vi "4461 - Create IO Channels Parallel.vi"(6 "error in":errorcluster, 7 "AI Buffer Size (S)":i32=10, 8 "sampling info":cluster{"Fs":dbl, "#s":dbl}, 9 "AO":T1={"AO amp (V)"=[0.1, 0.09, 0.08, 0.07, 0.06, 0.05, 0.04, 0.03], "AO DC (V)"=[0.0, 0.0, 0.0, 0.0, 0.0, 0.0, 0.0, 0.0], "AO f (Hz)"=[13.0, 13.0, 13.0, 13.0, 13.0, 13.0, 13.0, 13.0], "AO phi (deg)"=[0.0, 0.0, 0.0, 0.0, 0.0, 0.0, 0.0, 0.0], "function"=[enum."Sine Wave", enum."Sine Wave", enum."Sine Wave", enum."Sine Wave", enum."Sine Wave", enum."Sine Wave", enum."Sine Wave", enum."Sine Wave"]} {"AO DC (V)" format="%#_6p"; "AO amp (V)" format="%#_6p"}, 10 "AO Configuration":T2(array[cluster])=[{"Output physical channels"="PXI1Slot2/ao0", "AO. Max"=0.1, "AO.Min"=-0.1}, {"Output physical channels"="", "AO. Max"=0.1, "AO.Min"=-0.1}], 11 "AI Configuration":T3(array[cluster])=[{"AI.Coupling"=10050, "AI.Max"=10.0, "AI.Min"=-10.0, "Input physical channels"="PXI1Slot2/ai0:1"}, {"AI.Coupling"=10050, "AI.Max"=10.0, "AI.Min"=-10.0, "Input physical channels"="PXI1Slot3/ai0:3"}, {"AI.Coupling"=10050, "AI.Max"=10.0, "AI.Min"=-10.0, "Input physical channels"=""}] {"AI.Coupling" items=["AC"=10045, "DC"=10050, "GND"=10066]}) -> (2 "AO Task":refnum<k21>[](array[refnum]), 3 "AI task":refnum<k21>[](array[refnum]), 4 "error out":errorcluster, 5 "phase log":dbl[](array[numeric])=[0.99999999999938, 0.99999999999938])   [LabVIEW 2013]
uses:
  <vilib>/DAQmx/write.llb/DAQmx Write (Analog 1D Wfm NChan NSamp).vi
  <vilib>/DAQmx/create/channels.llb/DAQmx Create Channel (AO-Voltage-Basic).vi
  <vilib>/DAQmx/configure/timing.llb/DAQmx Timing (Sample Clock).vi
  <vilib>/DAQmx/create/channels.llb/DAQmx Create Channel (AI-Voltage-Basic).vi
  <vilib>/DAQmx/configure/trigger.llb/DAQmx Start Trigger (Digital Edge).vi
  <vilib>/DAQmx/miscellaneous.llb/DAQmx Fill In Error Info.vi
  <resource>/objmgr/daqmx.rc
panel:
  out "AI.Gain":dbl
  in  "input terminal configuration":i32(ring)=-1 items=["default"=-1, "RSE"=10083, "NRSE"=10078, "Differential"=10106, "Pseudodifferential"=12529]
  in  "output terminal configuration":i32(ring)=-1 items=["Default"=-1, "RSE"=10083, "Differential"=10106, "Pseudodifferential"=12529]
  out "SampClk.Timebase.Rate":dbl
  out "SampQuant.SampPerChan":dbl
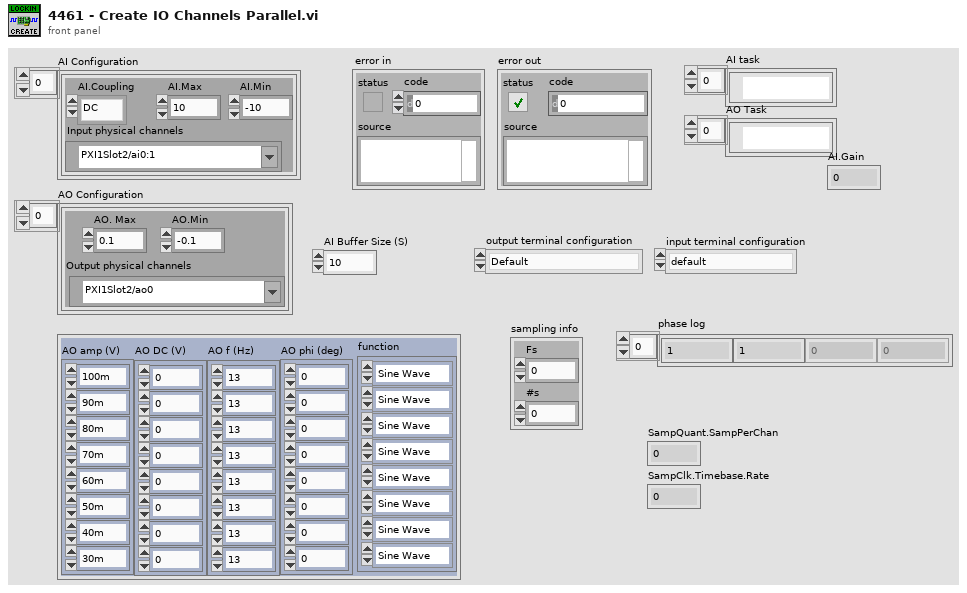
[diagram p1: front panel]
types:
  T1 = cluster{"AO amp (V)":dbl[], "AO DC (V)":dbl[], "AO f (Hz)":dbl[], "AO phi (deg)":dbl[], "function":enum16{"Sine Wave", "Triangle Wave", "Square Wave", "Sawtooth Wave"}[]}
  T2 = cluster{"Output physical channels":tag, "AO. Max":dbl, "AO.Min":dbl}[]
  T3 = cluster{"AI.Coupling":i32, "AI.Max":dbl, "AI.Min":dbl, "Input physical channels":tag}[]
  T4 = cluster{"AI.Coupling":i32, "AI.Max":dbl, "AI.Min":dbl, "Input physical channels":tag}
  T5 = cluster{"Output physical channels":tag, "AO. Max":dbl, "AO.Min":dbl}
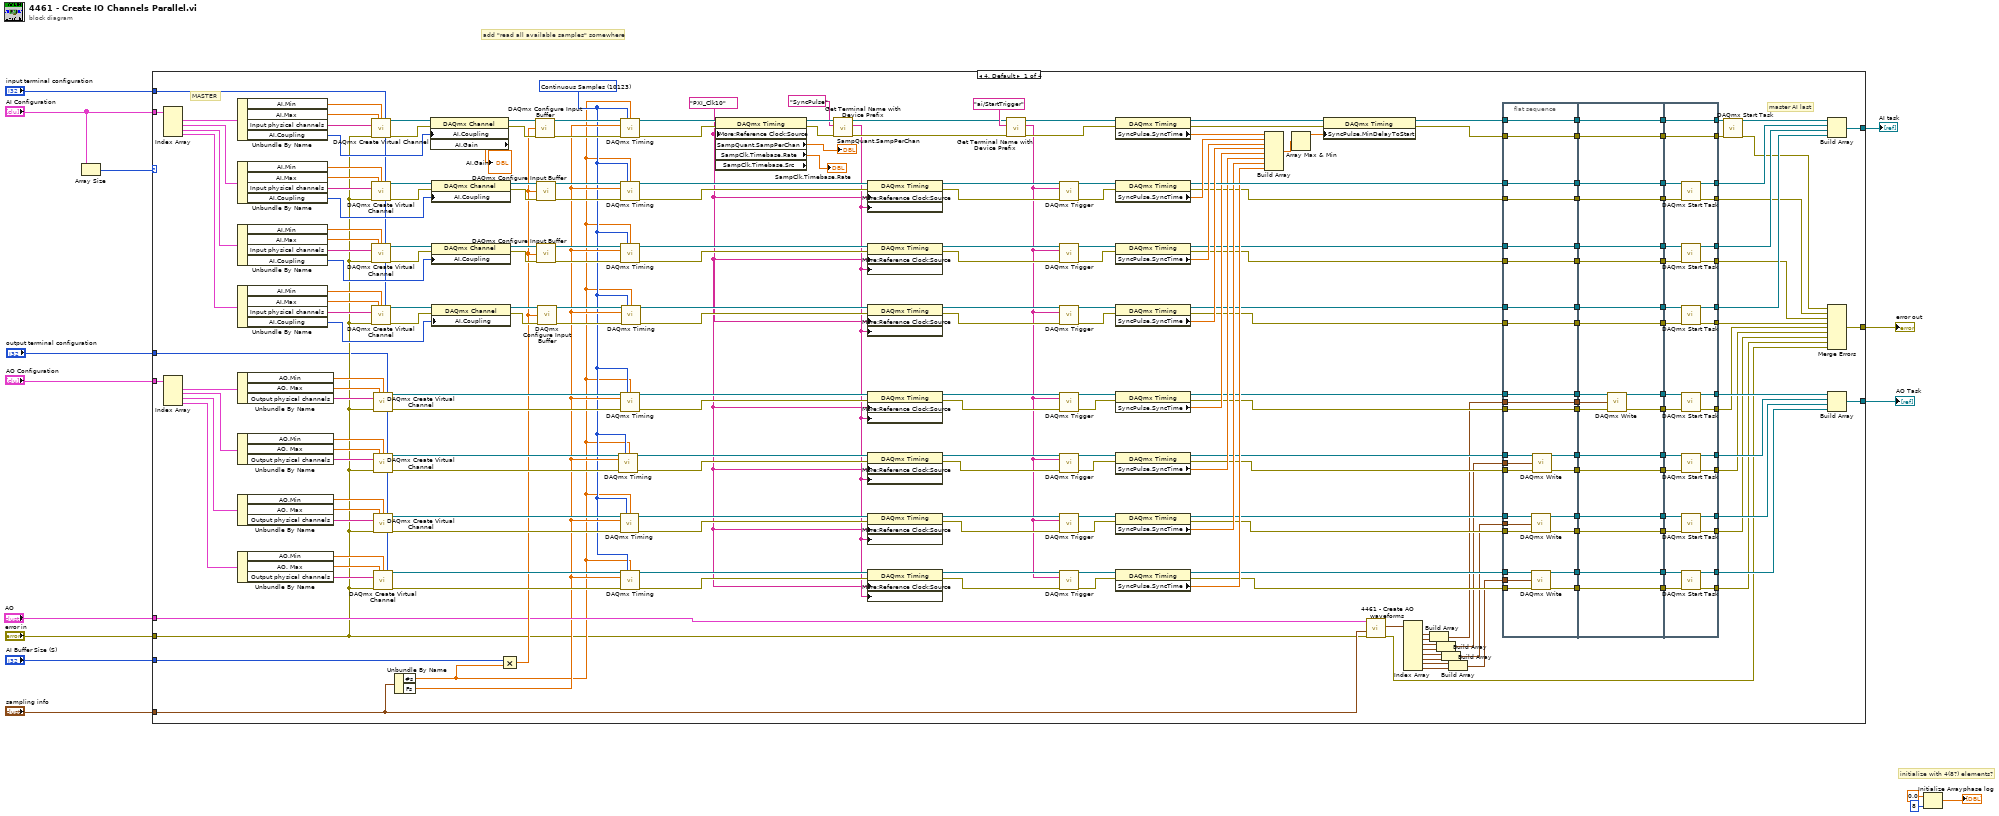
[diagram p0: block diagram]
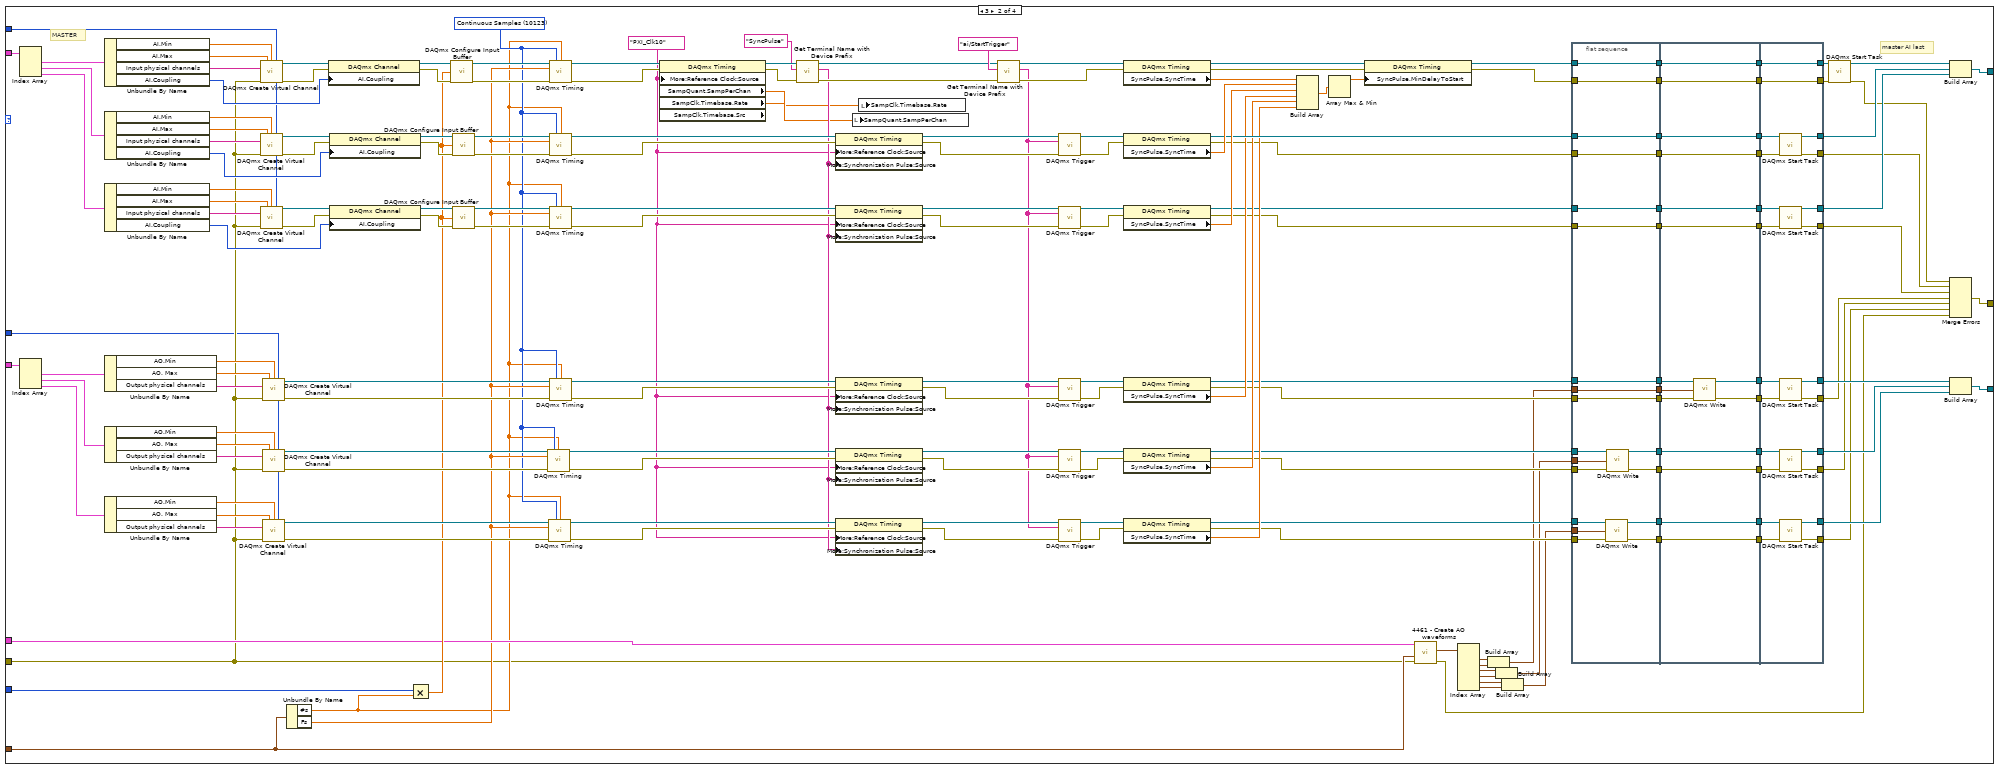
[diagram p2: hidden frame]
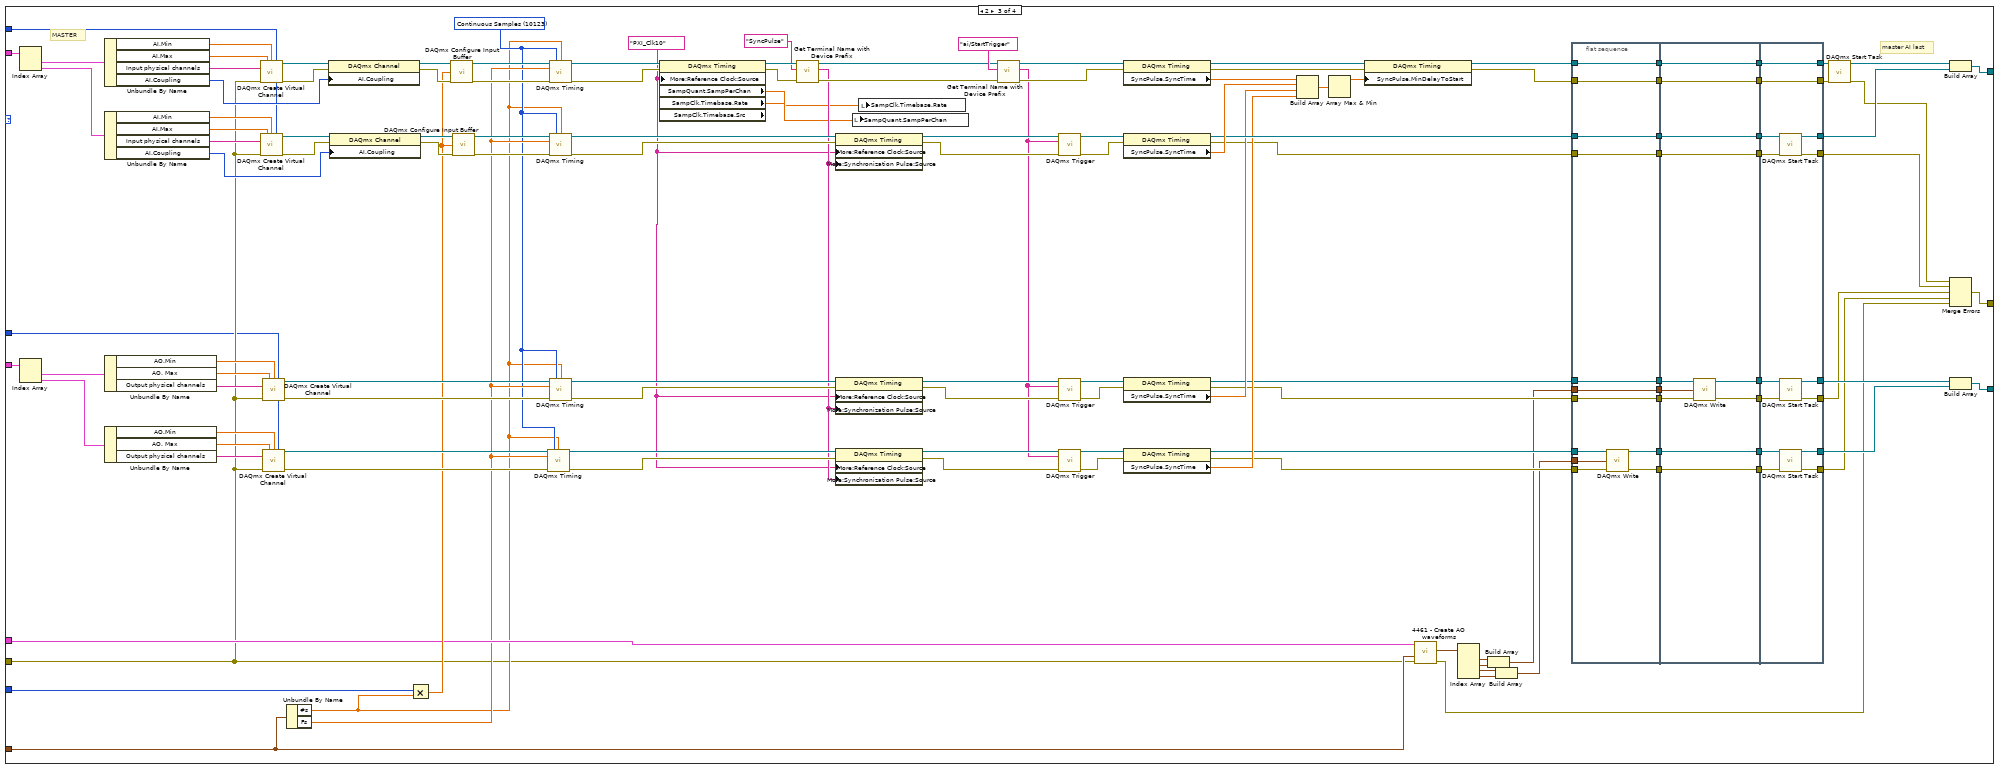
[diagram p3: hidden frame]
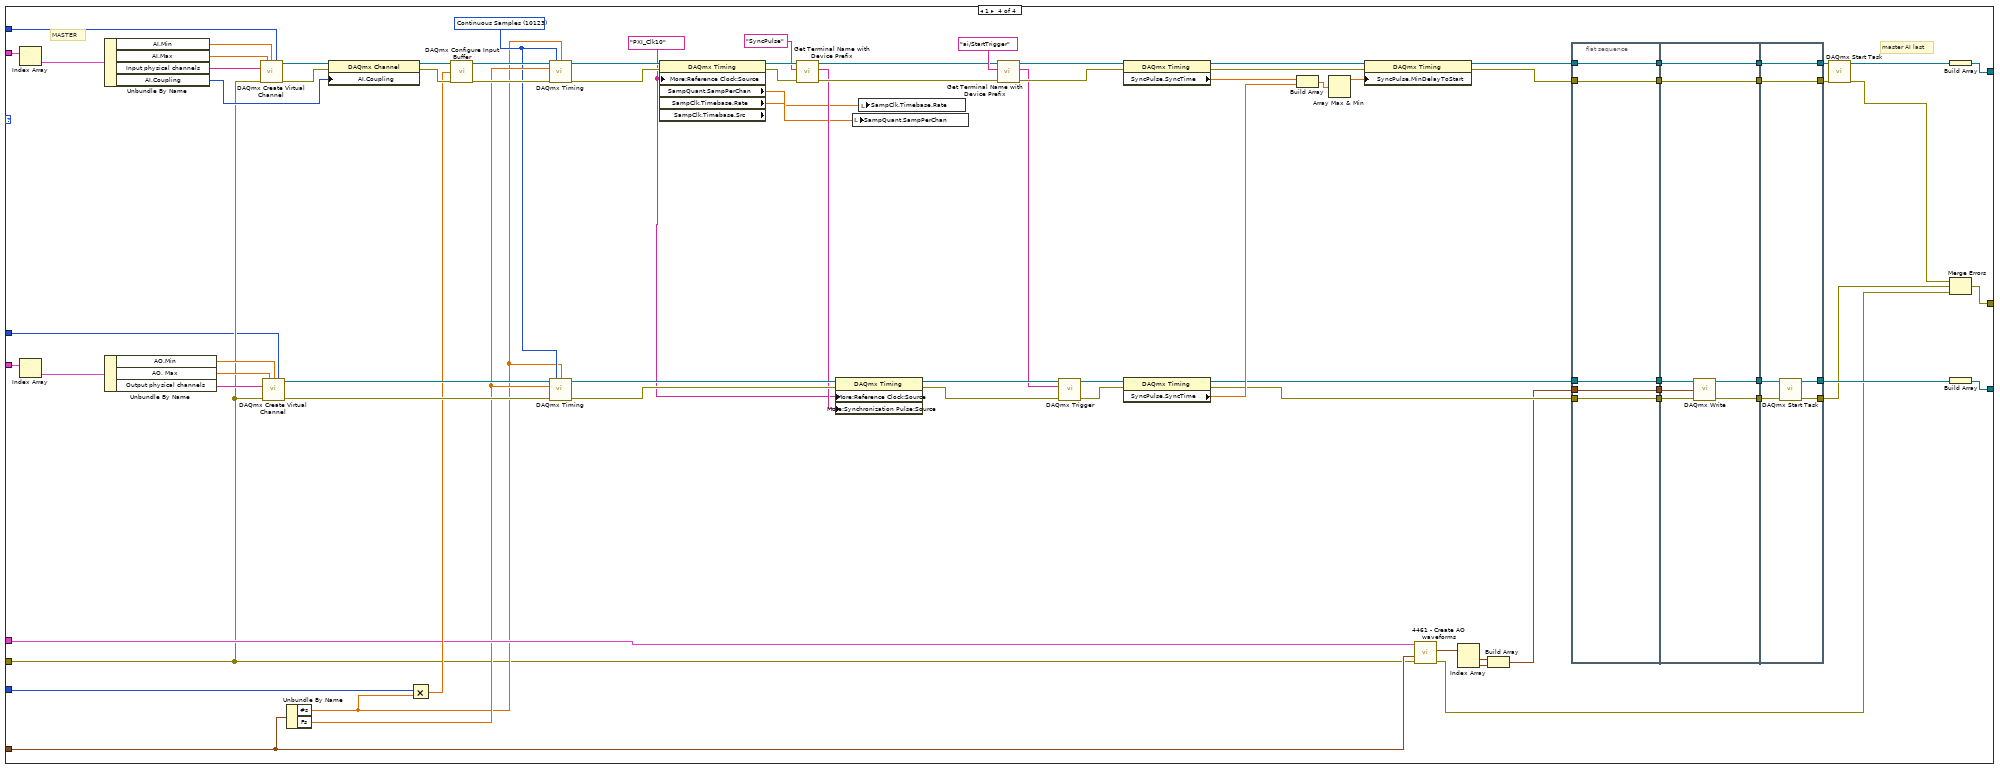
[diagram p4: hidden frame]
diagram:
  # "initialize with 4(8?) elements?"
  # "add \"read all available samples\" somewhere"
  n1 = Array Size(array="AI Configuration") -> (size(s)=w3:i32)
  n2 = case shown="4, Default" w3 {
    tunnel: "AI Buffer Size (S)" -> [w194 w460 w657 w785]
    tunnel: [w192 w458 w655 w783] -> w14
    tunnel: "AI Configuration" -> [w191 w457 w654 w782]
    tunnel: "AO Configuration" -> [w131 w414 w629 w776]
    tunnel: [w59 w361 w595 w760] -> w12
    tunnel: "AO" -> [w37 w343 w580 w748]
    tunnel: "sampling info" -> [w36 w342 w579 w747]
    tunnel: [w28 w335 w573 w742] -> w6
    tunnel: "error in" -> [w22 w330 w569 w739]
    tunnel: "output terminal configuration" -> [w17 w325 w565 w734]
    tunnel: "input terminal configuration" -> [w18 w326 w564 w735]
    frame 4, Default {
      w53 = tag "PXI_Clk10" ("RefClk.Src")
      w34 = 10123 items=["Finite Samples"=10178, "Continuous Samples"=10123] ("sample mode")
      # "master AI last"
      # "MASTER"
      n3 = Index Array(array=w191) -> (element #1=w216:T4, element #2=w178:T4, element #3=w144:T4, element #4=w143:T4)  [unwired: 4 in]
      n4 = Index Array(array=w131) -> (element #1=w130:T5, element #2=w85:T5, element #3=w86:T5, element #4=w87:T5)  [unwired: 4 in]
      n5 = Unbundle By Name(w216) -> ("AI.Min"=w189:dbl, "AI.Max"=w190:dbl, "Input physical channels"=w201:tag, "AI.Coupling"=w188:i32)
      n6 = Unbundle By Name(w178) -> ("AI.Min"=w185:dbl, "AI.Max"=w184:dbl, "Input physical channels"=w179:tag, "AI.Coupling"=w186:i32)
      n7 = Unbundle By Name(w144) -> ("AI.Min"=w159:dbl, "AI.Max"=w160:dbl, "Input physical channels"=w165:tag, "AI.Coupling"=w158:i32)
      n8 = Unbundle By Name(w143) -> ("AI.Min"=w156:dbl, "AI.Max"=w155:dbl, "Input physical channels"=w151:tag, "AI.Coupling"=w157:i32)
      n9 = Unbundle By Name(w130) -> ("AO.Min"=w127:dbl, "AO. Max"=w128:dbl, "Output physical channels"=w129:tag)
      n10 = Unbundle By Name(w85) -> ("AO.Min"=w112:dbl, "AO. Max"=w111:dbl, "Output physical channels"=w110:tag)
      n11 = Unbundle By Name(w86) -> ("AO.Min"=w107:dbl, "AO. Max"=w108:dbl, "Output physical channels"=w109:tag)
      n12 = Unbundle By Name(w87) -> ("AO.Min"=w90:dbl, "AO. Max"=w89:dbl, "Output physical channels"=w88:tag)
      n13 = call-poly <vilib>:"DAQmx Create Virtual Channel.vi"("maximum value"=w190, "minimum value"=w189, "input terminal configuration"=w18, "physical channels"=w201, "error in"=w22) -> ("task out"=w200:refnum<k21>, "error out"=w199:errorcluster)  [unwired: 9 in]
      n14 = call-poly <vilib>:"DAQmx Create Virtual Channel.vi"("maximum value"=w184, "minimum value"=w185, "input terminal configuration"=w18, "physical channels"=w179, "error in"=w22) -> ("task out"=w180:refnum<k21>, "error out"=w181:errorcluster)  [unwired: 9 in]
      n15 = call-poly <vilib>:"DAQmx Create Virtual Channel.vi"("maximum value"=w160, "minimum value"=w159, "input terminal configuration"=w18, "physical channels"=w165, "error in"=w22) -> ("task out"=w164:refnum<k21>, "error out"=w163:errorcluster)  [unwired: 9 in]
      n16 = call-poly <vilib>:"DAQmx Create Virtual Channel.vi"("maximum value"=w155, "minimum value"=w156, "input terminal configuration"=w18, "physical channels"=w151, "error in"=w22) -> ("task out"=w152:refnum<k21>, "error out"=w153:errorcluster)  [unwired: 9 in]
      n17 = call-poly <vilib>:"DAQmx Create Virtual Channel.vi"("maximum value"=w128, "minimum value"=w127, "output terminal configuration"=w17, "physical channels"=w129, "error in"=w22) -> ("task out"=w52:refnum<k21>, "error out"=w51:errorcluster)  [unwired: 9 in]
      n18 = call-poly <vilib>:"DAQmx Create Virtual Channel.vi"("maximum value"=w111, "minimum value"=w112, "output terminal configuration"=w17, "physical channels"=w110, "error in"=w22) -> ("task out"=w113:refnum<k21>, "error out"=w114:errorcluster)  [unwired: 9 in]
      n19 = call-poly <vilib>:"DAQmx Create Virtual Channel.vi"("maximum value"=w108, "minimum value"=w107, "output terminal configuration"=w17, "physical channels"=w109, "error in"=w22) -> ("task out"=w106:refnum<k21>, "error out"=w105:errorcluster)  [unwired: 9 in]
      n20 = call-poly <vilib>:"DAQmx Create Virtual Channel.vi"("maximum value"=w89, "minimum value"=w90, "output terminal configuration"=w17, "physical channels"=w88, "error in"=w22) -> ("task out"=w91:refnum<k21>, "error out"=w92:errorcluster)  [unwired: 9 in]
      n21 = Unbundle By Name(w36) -> ("#s"=w33:dbl, "Fs"=w35:dbl)
      n22 = property class="DAQmx Channel"(reference=w200, error in=w199, "AI.Coupling"=w188) -> (reference out=w198:refnum<k21>, error out=w197:errorcluster, "AI.Gain"=→"AI.Gain":dbl)
      n23 = property class="DAQmx Channel"(reference=w180, error in=w181, "AI.Coupling"=w186) -> (reference out=w182:refnum<k21>, error out=w183:errorcluster)
      n24 = property class="DAQmx Channel"(reference=w164, error in=w163, "AI.Coupling"=w158) -> (reference out=w162:refnum<k21>, error out=w161:errorcluster)
      n25 = property class="DAQmx Channel"(reference=w152, error in=w153, "AI.Coupling"=w157) -> (reference out=w154:refnum<k21>, error out=w58:errorcluster)
      n26 = Multiply(x=w194, y=w33) -> (x*y=w38:dbl)
      n27 = call <vilib>:"DAQmx Configure Input Buffer.vi"("task/channels in"=w198, "buffer size (in samples per channel)"=w38, "error in"=w197) -> ("task out"=w196:refnum<k21>, "error out"=w195:errorcluster)  [unwired: 11 in]
      n28 = call <vilib>:"DAQmx Configure Input Buffer.vi"("task/channels in"=w182, "buffer size (in samples per channel)"=w38, "error in"=w183) -> ("task out"=w177:refnum<k21>, "error out"=w176:errorcluster)  [unwired: 11 in]
      n29 = call <vilib>:"DAQmx Configure Input Buffer.vi"("task/channels in"=w162, "buffer size (in samples per channel)"=w38, "error in"=w161) -> ("task out"=w166:refnum<k21>, "error out"=w167:errorcluster)  [unwired: 11 in]
      n30 = call <vilib>:"DAQmx Configure Input Buffer.vi"("task/channels in"=w154, "buffer size (in samples per channel)"=w38, "error in"=w58) -> ("task out"=w150:refnum<k21>, "error out"=w149:errorcluster)  [unwired: 11 in]
      n31 = call-poly <vilib>:"DAQmx Timing.vi"("task/channels in"=w113, "sample mode"=w34, "samples per channel"=w33, "rate"=w35, "error in"=w114) -> ("task out"=w116:refnum<k21>, "error out"=w117:errorcluster)  [unwired: 9 in]
      n32 = call-poly <vilib>:"DAQmx Timing.vi"("task/channels in"=w106, "sample mode"=w34, "samples per channel"=w33, "rate"=w35, "error in"=w105) -> ("task out"=w103:refnum<k21>, "error out"=w102:errorcluster)  [unwired: 9 in]
      n33 = call-poly <vilib>:"DAQmx Timing.vi"("task/channels in"=w196, "sample mode"=w34, "samples per channel"=w33, "rate"=w35, "error in"=w195) -> ("task out"=w215:refnum<k21>, "error out"=w187:errorcluster)  [unwired: 9 in]
      n34 = call-poly <vilib>:"DAQmx Timing.vi"("task/channels in"=w177, "sample mode"=w34, "samples per channel"=w33, "rate"=w35, "error in"=w176) -> ("task out"=w175:refnum<k21>, "error out"=w174:errorcluster)  [unwired: 9 in]
      n35 = call-poly <vilib>:"DAQmx Timing.vi"("task/channels in"=w166, "sample mode"=w34, "samples per channel"=w33, "rate"=w35, "error in"=w167) -> ("task out"=w168:refnum<k21>, "error out"=w169:errorcluster)  [unwired: 9 in]
      n36 = call-poly <vilib>:"DAQmx Timing.vi"("task/channels in"=w52, "sample mode"=w34, "samples per channel"=w33, "rate"=w35, "error in"=w51) -> ("task out"=w125:refnum<k21>, "error out"=w124:errorcluster)  [unwired: 9 in]
      n37 = call-poly <vilib>:"DAQmx Timing.vi"("task/channels in"=w91, "sample mode"=w34, "samples per channel"=w33, "rate"=w35, "error in"=w92) -> ("task out"=w94:refnum<k21>, "error out"=w95:errorcluster)  [unwired: 9 in]
      n38 = call-poly <vilib>:"DAQmx Timing.vi"("task/channels in"=w150, "sample mode"=w34, "samples per channel"=w33, "rate"=w35, "error in"=w149) -> ("task out"=w148:refnum<k21>, "error out"=w147:errorcluster)  [unwired: 9 in]
      n39 = property class="DAQmx Timing" props=["More:Reference Clock:Source", "SampQuant.SampPerChan", "SampClk.Timebase.Rate", "SampClk.Timebase.Src"](reference=w215, error in=w187, "More:Reference Clock:Source"=w53) -> (reference out=w57:refnum<k21>, error out=w56:errorcluster, "SampQuant.SampPerChan"=→"SampQuant.SampPerChan":dbl, "SampClk.Timebase.Rate"=→"SampClk.Timebase.Rate":dbl)  [unwired: 1 out]
      n40 = call "Get Terminal Name with Device Prefix.vi"("error in (no error)"=w56, "Local Terminal Name"="SyncPulse", "task/channels in"=w57) -> ("error out"=w210:errorcluster, "Terminal Name with Device Prefix"=w54:tag, "task out"=w211:refnum<k21>)  [unwired: 6 in]
      n41 = property class="DAQmx Timing"(reference=w175, error in=w174, "More:Reference Clock:Source"=w53, "More:Synchronization Pulse:Source"=w54) -> (reference out=w173:refnum<k21>, error out=w172:errorcluster)
      n42 = property class="DAQmx Timing"(reference=w168, error in=w169, "More:Reference Clock:Source"=w53, "More:Synchronization Pulse:Source"=w54) -> (reference out=w170:refnum<k21>, error out=w171:errorcluster)
      n43 = property class="DAQmx Timing"(reference=w148, error in=w147, "More:Reference Clock:Source"=w53, "More:Synchronization Pulse:Source"=w54) -> (reference out=w146:refnum<k21>, error out=w145:errorcluster)
      n44 = property class="DAQmx Timing"(reference=w125, error in=w124, "More:Reference Clock:Source"=w53, "More:Synchronization Pulse:Source"=w54) -> (reference out=w126:refnum<k21>, error out=w123:errorcluster)
      n45 = property class="DAQmx Timing"(reference=w116, error in=w117, "More:Reference Clock:Source"=w53, "More:Synchronization Pulse:Source"=w54) -> (reference out=w115:refnum<k21>, error out=w118:errorcluster)
      n46 = property class="DAQmx Timing"(reference=w103, error in=w102, "More:Reference Clock:Source"=w53, "More:Synchronization Pulse:Source"=w54) -> (reference out=w104:refnum<k21>, error out=w101:errorcluster)
      n47 = property class="DAQmx Timing"(reference=w94, error in=w95, "More:Reference Clock:Source"=w53, "More:Synchronization Pulse:Source"=w54) -> (reference out=w93:refnum<k21>, error out=w96:errorcluster)
      n48 = call "Get Terminal Name with Device Prefix.vi"("error in (no error)"=w210, "Local Terminal Name"="ai/StartTrigger", "task/channels in"=w211) -> ("error out"=w208:errorcluster, "Terminal Name with Device Prefix"=w80:tag, "task out"=w209:refnum<k21>)  [unwired: 6 in]
      n49 = call-poly <vilib>:"DAQmx Trigger.vi"("task/channels in"=w173, "source"=w80, "error in"=w172) -> ("task out"=w140:refnum<k21>, "error out"=w139:errorcluster)  [unwired: 11 in]
      n50 = call-poly <vilib>:"DAQmx Trigger.vi"("task/channels in"=w170, "source"=w80, "error in"=w171) -> ("task out"=w141:refnum<k21>, "error out"=w138:errorcluster)  [unwired: 11 in]
      n51 = call-poly <vilib>:"DAQmx Trigger.vi"("task/channels in"=w146, "source"=w80, "error in"=w145) -> ("task out"=w142:refnum<k21>, "error out"=w137:errorcluster)  [unwired: 11 in]
      n52 = call-poly <vilib>:"DAQmx Trigger.vi"("task/channels in"=w126, "source"=w80, "error in"=w123) -> ("task out"=w122:refnum<k21>, "error out"=w121:errorcluster)  [unwired: 11 in]
      n53 = call-poly <vilib>:"DAQmx Trigger.vi"("task/channels in"=w115, "source"=w80, "error in"=w118) -> ("task out"=w119:refnum<k21>, "error out"=w120:errorcluster)  [unwired: 11 in]
      n54 = call-poly <vilib>:"DAQmx Trigger.vi"("task/channels in"=w104, "source"=w80, "error in"=w101) -> ("task out"=w100:refnum<k21>, "error out"=w99:errorcluster)  [unwired: 11 in]
      n55 = call-poly <vilib>:"DAQmx Trigger.vi"("task/channels in"=w93, "source"=w80, "error in"=w96) -> ("task out"=w97:refnum<k21>, "error out"=w98:errorcluster)  [unwired: 11 in]
      n56 = property class="DAQmx Timing"(reference=w209, error in=w208) -> (reference out=w205:refnum<k21>, error out=w206:errorcluster, "SyncPulse.SyncTime"=w207:dbl)
      n57 = property class="DAQmx Timing"(reference=w140, error in=w139) -> (reference out=w132:refnum<k21>, error out=w77:errorcluster, "SyncPulse.SyncTime"=w135:dbl)
      n58 = property class="DAQmx Timing"(reference=w141, error in=w138) -> (reference out=w79:refnum<k21>, error out=w76:errorcluster, "SyncPulse.SyncTime"=w134:dbl)
      n59 = property class="DAQmx Timing"(reference=w142, error in=w137) -> (reference out=w78:refnum<k21>, error out=w75:errorcluster, "SyncPulse.SyncTime"=w133:dbl)
      n60 = property class="DAQmx Timing"(reference=w122, error in=w121) -> (reference out=w74:refnum<k21>, error out=w71:errorcluster, "SyncPulse.SyncTime"=w84:dbl)
      n61 = property class="DAQmx Timing"(reference=w119, error in=w120) -> (reference out=w73:refnum<k21>, error out=w70:errorcluster, "SyncPulse.SyncTime"=w83:dbl)
      n62 = property class="DAQmx Timing"(reference=w100, error in=w99) -> (reference out=w72:refnum<k21>, error out=w69:errorcluster, "SyncPulse.SyncTime"=w82:dbl)
      n63 = property class="DAQmx Timing"(reference=w97, error in=w98) -> (reference out=w68:refnum<k21>, error out=w67:errorcluster, "SyncPulse.SyncTime"=w81:dbl)
      n64 = Build Array(w207, w135, w134, w133, w84, w83, w82, w81) -> (w204:dbl[])
      n65 = Array Max & Min(array=w204) -> (max value=w136:dbl)  [unwired: 3 out]
      n66 = property class="DAQmx Timing"(reference=w205, error in=w206, "SyncPulse.MinDelayToStart"=w136) -> (reference out=w202:refnum<k21>, error out=w203:errorcluster)
      n67 = call "4461 - Create AO waveforms.vi"("error in (no error)"=w22, "sampling info"=w36, "AO"=w37) -> ("error out"=w21:errorcluster, "AO Array"=w23:waveform(dbl)[])  [unwired: 5 in, 2 out]
      n68 = Index Array(array=w23) -> (element #1=w39:waveform(dbl), element #2=w50:waveform(dbl), element #3=w49:waveform(dbl), element #4=w48:waveform(dbl), element #5=w47:waveform(dbl), element #6=w46:waveform(dbl), element #7=w45:waveform(dbl), element #8=w44:waveform(dbl))  [unwired: 8 in]
      n69 = Build Array(w39, w50) -> (w43:waveform(dbl)[])
      n70 = Build Array(w49, w48) -> (w42:waveform(dbl)[])
      n71 = Build Array(w47, w46) -> (w41:waveform(dbl)[])
      n72 = Build Array(w45, w44) -> (w40:waveform(dbl)[])
      n73 = flat-sequence {
        tunnel: w203 -> [w274]
        tunnel: w202 -> [w275]
        tunnel: [w275] -> w249
        tunnel: [w274] -> w248
        tunnel: [w273] -> w247
        tunnel: w132 -> [w273]
        tunnel: [w272] -> w246
        tunnel: w79 -> [w272]
        tunnel: [w271] -> w245
        tunnel: w78 -> [w271]
        tunnel: [w270] -> w244
        tunnel: w77 -> [w270]
        tunnel: [w269] -> w243
        tunnel: w76 -> [w269]
        tunnel: [w268] -> w242
        tunnel: w75 -> [w268]
        tunnel: [w267] -> w241
        tunnel: w74 -> [w267]
        tunnel: [w255] -> w240
        tunnel: w73 -> [w256]
        tunnel: [w259] -> w239
        tunnel: w72 -> [w258]
        tunnel: [w266] -> w238
        tunnel: w71 -> [w266]
        tunnel: w70 -> [w257]
        tunnel: [w260] -> w237
        tunnel: w69 -> [w261]
        tunnel: [w262] -> w236
        tunnel: w68 -> [w265]
        tunnel: [w263] -> w235
        tunnel: w67 -> [w264]
        tunnel: [w254] -> w234
        tunnel: [w253] -> w233
        tunnel: w43 -> [w253]
        tunnel: w42 -> [w252]
        tunnel: w41 -> [w251]
        tunnel: w40 -> [w250]
        tunnel: [w294] -> w232
        tunnel: [w293] -> w231
        tunnel: w249 -> [w294]
        tunnel: w248 -> [w293]
        tunnel: [w292] -> w230
        tunnel: w247 -> [w292]
        tunnel: [w291] -> w229
        tunnel: w246 -> [w291]
        tunnel: [w290] -> w228
        tunnel: w245 -> [w290]
        tunnel: [w289] -> w227
        tunnel: w244 -> [w289]
        tunnel: [w288] -> w226
        tunnel: w243 -> [w288]
        tunnel: [w287] -> w225
        tunnel: w242 -> [w287]
        tunnel: [w279] -> w224
        tunnel: w241 -> [w280]
        tunnel: [w286] -> w223
        tunnel: w240 -> [w286]
        tunnel: [w285] -> w222
        tunnel: w239 -> [w285]
        tunnel: [w278] -> w221
        tunnel: w238 -> [w277]
        tunnel: [w284] -> w220
        tunnel: [w283] -> w219
        tunnel: w237 -> [w283]
        tunnel: [w282] -> w218
        tunnel: w236 -> [w282]
        tunnel: [w281] -> w217
        tunnel: w235 -> [w281]
        tunnel: w234 -> [w284]
        tunnel: w233 -> [w276]
        tunnel: [w324] -> w214
        tunnel: [w323] -> w213
        tunnel: w232 -> [w324]
        tunnel: w231 -> [w323]
        tunnel: w230 -> [w322]
        tunnel: w229 -> [w321]
        tunnel: w228 -> [w320]
        tunnel: w227 -> [w319]
        tunnel: w226 -> [w318]
        tunnel: w225 -> [w317]
        tunnel: w224 -> [w316]
        tunnel: w223 -> [w315]
        tunnel: w222 -> [w314]
        tunnel: w221 -> [w313]
        tunnel: w220 -> [w312]
        tunnel: w219 -> [w311]
        tunnel: w218 -> [w310]
        tunnel: w217 -> [w309]
        tunnel: [w308] -> w66
        tunnel: [w307] -> w65
        tunnel: [w306] -> w64
        tunnel: [w305] -> w63
        tunnel: [w304] -> w62
        tunnel: [w303] -> w61
        tunnel: [w302] -> w60
        tunnel: [w301] -> w31
        tunnel: [w300] -> w30
        tunnel: [w299] -> w29
        tunnel: [w298] -> w27
        tunnel: [w297] -> w26
        tunnel: [w296] -> w25
        tunnel: [w295] -> w24
        frame #0 {
          n74 = call-poly <vilib>:"DAQmx Write.vi"("task/channels in"=w258, "data"=w251, "error in"=w261) -> ("task out"=w259:refnum<k21>, "error out"=w260:errorcluster)  [unwired: 10 in, 1 out]
          n75 = call-poly <vilib>:"DAQmx Write.vi"("task/channels in"=w265, "data"=w250, "error in"=w264) -> ("task out"=w262:refnum<k21>, "error out"=w263:errorcluster)  [unwired: 10 in, 1 out]
          n76 = call-poly <vilib>:"DAQmx Write.vi"("task/channels in"=w256, "data"=w252, "error in"=w257) -> ("task out"=w255:refnum<k21>, "error out"=w254:errorcluster)  [unwired: 10 in, 1 out]
        }
        frame #1 {
          n77 = call-poly <vilib>:"DAQmx Write.vi"("task/channels in"=w280, "data"=w276, "error in"=w277) -> ("task out"=w279:refnum<k21>, "error out"=w278:errorcluster)  [unwired: 10 in, 1 out]
        }
        frame #2 {
          n78 = call <vilib>:"DAQmx Start Task.vi"("task/channels in"=w322, "error in"=w319) -> ("task out"=w308:refnum<k21>, "error out"=w301:errorcluster)  [unwired: 12 in]
          n79 = call <vilib>:"DAQmx Start Task.vi"("task/channels in"=w321, "error in"=w318) -> ("task out"=w307:refnum<k21>, "error out"=w300:errorcluster)  [unwired: 12 in]
          n80 = call <vilib>:"DAQmx Start Task.vi"("task/channels in"=w320, "error in"=w317) -> ("task out"=w306:refnum<k21>, "error out"=w299:errorcluster)  [unwired: 12 in]
          n81 = call <vilib>:"DAQmx Start Task.vi"("task/channels in"=w316, "error in"=w313) -> ("task out"=w305:refnum<k21>, "error out"=w298:errorcluster)  [unwired: 12 in]
          n82 = call <vilib>:"DAQmx Start Task.vi"("task/channels in"=w315, "error in"=w312) -> ("task out"=w304:refnum<k21>, "error out"=w297:errorcluster)  [unwired: 12 in]
          n83 = call <vilib>:"DAQmx Start Task.vi"("task/channels in"=w314, "error in"=w311) -> ("task out"=w303:refnum<k21>, "error out"=w296:errorcluster)  [unwired: 12 in]
          n84 = call <vilib>:"DAQmx Start Task.vi"("task/channels in"=w310, "error in"=w309) -> ("task out"=w302:refnum<k21>, "error out"=w295:errorcluster)  [unwired: 12 in]
        }
      }
      n85 = call <vilib>:"DAQmx Start Task.vi"("task/channels in"=w214, "error in"=w213) -> ("task out"=w193:refnum<k21>, "error out"=w32:errorcluster)  [unwired: 12 in]
      n86 = Build Array(w193, w66, w65, w64) -> (w192:refnum<k21>[])
      n87 = Merge Errors(w32, w31, w30, w29, w27, w26, w25, w24, w21) -> (w28:errorcluster)
      n88 = Build Array(w63, w62, w61, w60) -> (w59:refnum<k21>[])
    }
    frame 3 {
      w356 = tag "PXI_Clk10" ("RefClk.Src")
      w340 = 10123 items=["Finite Samples"=10178, "Continuous Samples"=10123] ("sample mode")
      # "master AI last"
      # "MASTER"
      n89 = Index Array(array=w457) -> (element #1=w482:T4, element #2=w444:T4, element #3=w423:T4)  [unwired: 3 in]
      n90 = Index Array(array=w414) -> (element #1=w413:T5, element #2=w380:T5, element #3=w381:T5)  [unwired: 3 in]
      n91 = Unbundle By Name(w482) -> ("AI.Min"=w455:dbl, "AI.Max"=w456:dbl, "Input physical channels"=w467:tag, "AI.Coupling"=w454:i32)
      n92 = Unbundle By Name(w444) -> ("AI.Min"=w451:dbl, "AI.Max"=w450:dbl, "Input physical channels"=w445:tag, "AI.Coupling"=w452:i32)
      n93 = Unbundle By Name(w423) -> ("AI.Min"=w425:dbl, "AI.Max"=w426:dbl, "Input physical channels"=w431:tag, "AI.Coupling"=w424:i32)
      n94 = Unbundle By Name(w413) -> ("AO.Min"=w410:dbl, "AO. Max"=w411:dbl, "Output physical channels"=w412:tag)
      n95 = Unbundle By Name(w380) -> ("AO.Min"=w395:dbl, "AO. Max"=w394:dbl, "Output physical channels"=w393:tag)
      n96 = Unbundle By Name(w381) -> ("AO.Min"=w390:dbl, "AO. Max"=w391:dbl, "Output physical channels"=w392:tag)
      n97 = call-poly <vilib>:"DAQmx Create Virtual Channel.vi"("maximum value"=w456, "minimum value"=w455, "input terminal configuration"=w326, "physical channels"=w467, "error in"=w330) -> ("task out"=w466:refnum<k21>, "error out"=w465:errorcluster)  [unwired: 9 in]
      n98 = call-poly <vilib>:"DAQmx Create Virtual Channel.vi"("maximum value"=w450, "minimum value"=w451, "input terminal configuration"=w326, "physical channels"=w445, "error in"=w330) -> ("task out"=w446:refnum<k21>, "error out"=w447:errorcluster)  [unwired: 9 in]
      n99 = call-poly <vilib>:"DAQmx Create Virtual Channel.vi"("maximum value"=w426, "minimum value"=w425, "input terminal configuration"=w326, "physical channels"=w431, "error in"=w330) -> ("task out"=w430:refnum<k21>, "error out"=w429:errorcluster)  [unwired: 9 in]
      n100 = call-poly <vilib>:"DAQmx Create Virtual Channel.vi"("maximum value"=w411, "minimum value"=w410, "output terminal configuration"=w325, "physical channels"=w412, "error in"=w330) -> ("task out"=w355:refnum<k21>, "error out"=w354:errorcluster)  [unwired: 9 in]
      n101 = call-poly <vilib>:"DAQmx Create Virtual Channel.vi"("maximum value"=w394, "minimum value"=w395, "output terminal configuration"=w325, "physical channels"=w393, "error in"=w330) -> ("task out"=w396:refnum<k21>, "error out"=w397:errorcluster)  [unwired: 9 in]
      n102 = call-poly <vilib>:"DAQmx Create Virtual Channel.vi"("maximum value"=w391, "minimum value"=w390, "output terminal configuration"=w325, "physical channels"=w392, "error in"=w330) -> ("task out"=w389:refnum<k21>, "error out"=w388:errorcluster)  [unwired: 9 in]
      n103 = Unbundle By Name(w342) -> ("#s"=w339:dbl, "Fs"=w341:dbl)
      n104 = property class="DAQmx Channel"(reference=w466, error in=w465, "AI.Coupling"=w454) -> (reference out=w464:refnum<k21>, error out=w463:errorcluster)
      n105 = property class="DAQmx Channel"(reference=w446, error in=w447, "AI.Coupling"=w452) -> (reference out=w448:refnum<k21>, error out=w449:errorcluster)
      n106 = property class="DAQmx Channel"(reference=w430, error in=w429, "AI.Coupling"=w424) -> (reference out=w428:refnum<k21>, error out=w427:errorcluster)
      n107 = Multiply(x=w460, y=w339) -> (x*y=w344:dbl)
      n108 = call <vilib>:"DAQmx Configure Input Buffer.vi"("task/channels in"=w464, "buffer size (in samples per channel)"=w344, "error in"=w463) -> ("task out"=w462:refnum<k21>, "error out"=w461:errorcluster)  [unwired: 11 in]
      n109 = call <vilib>:"DAQmx Configure Input Buffer.vi"("task/channels in"=w448, "buffer size (in samples per channel)"=w344, "error in"=w449) -> ("task out"=w443:refnum<k21>, "error out"=w442:errorcluster)  [unwired: 11 in]
      n110 = call <vilib>:"DAQmx Configure Input Buffer.vi"("task/channels in"=w428, "buffer size (in samples per channel)"=w344, "error in"=w427) -> ("task out"=w432:refnum<k21>, "error out"=w433:errorcluster)  [unwired: 11 in]
      n111 = call-poly <vilib>:"DAQmx Timing.vi"("task/channels in"=w396, "sample mode"=w340, "samples per channel"=w339, "rate"=w341, "error in"=w397) -> ("task out"=w399:refnum<k21>, "error out"=w400:errorcluster)  [unwired: 9 in]
      n112 = call-poly <vilib>:"DAQmx Timing.vi"("task/channels in"=w389, "sample mode"=w340, "samples per channel"=w339, "rate"=w341, "error in"=w388) -> ("task out"=w386:refnum<k21>, "error out"=w385:errorcluster)  [unwired: 9 in]
      n113 = call-poly <vilib>:"DAQmx Timing.vi"("task/channels in"=w462, "sample mode"=w340, "samples per channel"=w339, "rate"=w341, "error in"=w461) -> ("task out"=w481:refnum<k21>, "error out"=w453:errorcluster)  [unwired: 9 in]
      n114 = call-poly <vilib>:"DAQmx Timing.vi"("task/channels in"=w443, "sample mode"=w340, "samples per channel"=w339, "rate"=w341, "error in"=w442) -> ("task out"=w441:refnum<k21>, "error out"=w440:errorcluster)  [unwired: 9 in]
      n115 = call-poly <vilib>:"DAQmx Timing.vi"("task/channels in"=w432, "sample mode"=w340, "samples per channel"=w339, "rate"=w341, "error in"=w433) -> ("task out"=w434:refnum<k21>, "error out"=w435:errorcluster)  [unwired: 9 in]
      n116 = call-poly <vilib>:"DAQmx Timing.vi"("task/channels in"=w355, "sample mode"=w340, "samples per channel"=w339, "rate"=w341, "error in"=w354) -> ("task out"=w408:refnum<k21>, "error out"=w407:errorcluster)  [unwired: 9 in]
      n117 = property class="DAQmx Timing" props=["More:Reference Clock:Source", "SampQuant.SampPerChan", "SampClk.Timebase.Rate", "SampClk.Timebase.Src"](reference=w481, error in=w453, "More:Reference Clock:Source"=w356) -> (reference out=w360:refnum<k21>, error out=w359:errorcluster, "SampQuant.SampPerChan"=w328:dbl, "SampClk.Timebase.Rate"=w327:dbl)  [unwired: 1 out]
      n118 = call "Get Terminal Name with Device Prefix.vi"("error in (no error)"=w359, "Local Terminal Name"="SyncPulse", "task/channels in"=w360) -> ("error out"=w476:errorcluster, "Terminal Name with Device Prefix"=w357:tag, "task out"=w477:refnum<k21>)  [unwired: 6 in]
      n119 = property class="DAQmx Timing"(reference=w441, error in=w440, "More:Reference Clock:Source"=w356, "More:Synchronization Pulse:Source"=w357) -> (reference out=w439:refnum<k21>, error out=w438:errorcluster)
      n120 = property class="DAQmx Timing"(reference=w434, error in=w435, "More:Reference Clock:Source"=w356, "More:Synchronization Pulse:Source"=w357) -> (reference out=w436:refnum<k21>, error out=w437:errorcluster)
      n121 = property class="DAQmx Timing"(reference=w408, error in=w407, "More:Reference Clock:Source"=w356, "More:Synchronization Pulse:Source"=w357) -> (reference out=w409:refnum<k21>, error out=w406:errorcluster)
      n122 = property class="DAQmx Timing"(reference=w399, error in=w400, "More:Reference Clock:Source"=w356, "More:Synchronization Pulse:Source"=w357) -> (reference out=w398:refnum<k21>, error out=w401:errorcluster)
      n123 = property class="DAQmx Timing"(reference=w386, error in=w385, "More:Reference Clock:Source"=w356, "More:Synchronization Pulse:Source"=w357) -> (reference out=w387:refnum<k21>, error out=w384:errorcluster)
      n124 = local write "SampQuant.SampPerChan"(w328) -> ()
      n125 = local write "SampClk.Timebase.Rate"(w327) -> ()
      n126 = call "Get Terminal Name with Device Prefix.vi"("error in (no error)"=w476, "Local Terminal Name"="ai/StartTrigger", "task/channels in"=w477) -> ("error out"=w474:errorcluster, "Terminal Name with Device Prefix"=w376:tag, "task out"=w475:refnum<k21>)  [unwired: 6 in]
      n127 = call-poly <vilib>:"DAQmx Trigger.vi"("task/channels in"=w439, "source"=w376, "error in"=w438) -> ("task out"=w421:refnum<k21>, "error out"=w420:errorcluster)  [unwired: 11 in]
      n128 = call-poly <vilib>:"DAQmx Trigger.vi"("task/channels in"=w436, "source"=w376, "error in"=w437) -> ("task out"=w422:refnum<k21>, "error out"=w419:errorcluster)  [unwired: 11 in]
      n129 = call-poly <vilib>:"DAQmx Trigger.vi"("task/channels in"=w409, "source"=w376, "error in"=w406) -> ("task out"=w405:refnum<k21>, "error out"=w404:errorcluster)  [unwired: 11 in]
      n130 = call-poly <vilib>:"DAQmx Trigger.vi"("task/channels in"=w398, "source"=w376, "error in"=w401) -> ("task out"=w402:refnum<k21>, "error out"=w403:errorcluster)  [unwired: 11 in]
      n131 = call-poly <vilib>:"DAQmx Trigger.vi"("task/channels in"=w387, "source"=w376, "error in"=w384) -> ("task out"=w383:refnum<k21>, "error out"=w382:errorcluster)  [unwired: 11 in]
      n132 = property class="DAQmx Timing"(reference=w475, error in=w474) -> (reference out=w471:refnum<k21>, error out=w472:errorcluster, "SyncPulse.SyncTime"=w473:dbl)
      n133 = property class="DAQmx Timing"(reference=w421, error in=w420) -> (reference out=w415:refnum<k21>, error out=w374:errorcluster, "SyncPulse.SyncTime"=w417:dbl)
      n134 = property class="DAQmx Timing"(reference=w422, error in=w419) -> (reference out=w375:refnum<k21>, error out=w373:errorcluster, "SyncPulse.SyncTime"=w416:dbl)
      n135 = property class="DAQmx Timing"(reference=w405, error in=w404) -> (reference out=w372:refnum<k21>, error out=w369:errorcluster, "SyncPulse.SyncTime"=w379:dbl)
      n136 = property class="DAQmx Timing"(reference=w402, error in=w403) -> (reference out=w371:refnum<k21>, error out=w368:errorcluster, "SyncPulse.SyncTime"=w378:dbl)
      n137 = property class="DAQmx Timing"(reference=w383, error in=w382) -> (reference out=w370:refnum<k21>, error out=w367:errorcluster, "SyncPulse.SyncTime"=w377:dbl)
      n138 = Build Array(w473, w417, w416, w379, w378, w377) -> (w470:dbl[])
      n139 = Array Max & Min(array=w470) -> (max value=w418:dbl)  [unwired: 3 out]
      n140 = property class="DAQmx Timing"(reference=w471, error in=w472, "SyncPulse.MinDelayToStart"=w418) -> (reference out=w468:refnum<k21>, error out=w469:errorcluster)
      n141 = call "4461 - Create AO waveforms.vi"("error in (no error)"=w330, "sampling info"=w342, "AO"=w343) -> ("error out"=w329:errorcluster, "AO Array"=w331:waveform(dbl)[])  [unwired: 5 in, 2 out]
      n142 = Index Array(array=w331) -> (element #1=w345:waveform(dbl), element #2=w353:waveform(dbl), element #3=w352:waveform(dbl), element #4=w351:waveform(dbl), element #5=w350:waveform(dbl), element #6=w349:waveform(dbl))  [unwired: 6 in]
      n143 = Build Array(w345, w353) -> (w348:waveform(dbl)[])
      n144 = Build Array(w352, w351) -> (w347:waveform(dbl)[])
      n145 = Build Array(w350, w349) -> (w346:waveform(dbl)[])
      n146 = flat-sequence {
        tunnel: w469 -> [w525]
        tunnel: w468 -> [w526]
        tunnel: [w526] -> w507
        tunnel: [w525] -> w506
        tunnel: [w524] -> w505
        tunnel: w415 -> [w524]
        tunnel: [w523] -> w504
        tunnel: w375 -> [w523]
        tunnel: [w522] -> w503
        tunnel: w374 -> [w522]
        tunnel: [w521] -> w502
        tunnel: w373 -> [w521]
        tunnel: [w520] -> w501
        tunnel: w372 -> [w520]
        tunnel: [w512] -> w500
        tunnel: w371 -> [w513]
        tunnel: [w516] -> w499
        tunnel: w370 -> [w515]
        tunnel: [w519] -> w498
        tunnel: w369 -> [w519]
        tunnel: w368 -> [w514]
        tunnel: [w517] -> w497
        tunnel: w367 -> [w518]
        tunnel: [w511] -> w496
        tunnel: [w510] -> w495
        tunnel: w348 -> [w510]
        tunnel: w347 -> [w509]
        tunnel: w346 -> [w508]
        tunnel: [w541] -> w494
        tunnel: [w540] -> w493
        tunnel: w507 -> [w541]
        tunnel: w506 -> [w540]
        tunnel: [w539] -> w492
        tunnel: w505 -> [w539]
        tunnel: [w538] -> w491
        tunnel: w504 -> [w538]
        tunnel: [w537] -> w490
        tunnel: w503 -> [w537]
        tunnel: [w536] -> w489
        tunnel: w502 -> [w536]
        tunnel: [w530] -> w488
        tunnel: w501 -> [w531]
        tunnel: [w535] -> w487
        tunnel: w500 -> [w535]
        tunnel: [w534] -> w486
        tunnel: w499 -> [w534]
        tunnel: [w529] -> w485
        tunnel: w498 -> [w528]
        tunnel: [w533] -> w484
        tunnel: [w532] -> w483
        tunnel: w497 -> [w532]
        tunnel: w496 -> [w533]
        tunnel: w495 -> [w527]
        tunnel: [w563] -> w480
        tunnel: [w562] -> w479
        tunnel: w494 -> [w563]
        tunnel: w493 -> [w562]
        tunnel: w492 -> [w561]
        tunnel: w491 -> [w560]
        tunnel: w490 -> [w559]
        tunnel: w489 -> [w558]
        tunnel: w488 -> [w557]
        tunnel: w487 -> [w556]
        tunnel: w486 -> [w555]
        tunnel: w485 -> [w554]
        tunnel: w484 -> [w553]
        tunnel: w483 -> [w552]
        tunnel: [w551] -> w366
        tunnel: [w550] -> w365
        tunnel: [w549] -> w364
        tunnel: [w548] -> w363
        tunnel: [w547] -> w362
        tunnel: [w546] -> w337
        tunnel: [w545] -> w336
        tunnel: [w544] -> w334
        tunnel: [w543] -> w333
        tunnel: [w542] -> w332
        frame #0 {
          n147 = call-poly <vilib>:"DAQmx Write.vi"("task/channels in"=w515, "data"=w508, "error in"=w518) -> ("task out"=w516:refnum<k21>, "error out"=w517:errorcluster)  [unwired: 10 in, 1 out]
          n148 = call-poly <vilib>:"DAQmx Write.vi"("task/channels in"=w513, "data"=w509, "error in"=w514) -> ("task out"=w512:refnum<k21>, "error out"=w511:errorcluster)  [unwired: 10 in, 1 out]
        }
        frame #1 {
          n149 = call-poly <vilib>:"DAQmx Write.vi"("task/channels in"=w531, "data"=w527, "error in"=w528) -> ("task out"=w530:refnum<k21>, "error out"=w529:errorcluster)  [unwired: 10 in, 1 out]
        }
        frame #2 {
          n150 = call <vilib>:"DAQmx Start Task.vi"("task/channels in"=w561, "error in"=w559) -> ("task out"=w551:refnum<k21>, "error out"=w546:errorcluster)  [unwired: 12 in]
          n151 = call <vilib>:"DAQmx Start Task.vi"("task/channels in"=w560, "error in"=w558) -> ("task out"=w550:refnum<k21>, "error out"=w545:errorcluster)  [unwired: 12 in]
          n152 = call <vilib>:"DAQmx Start Task.vi"("task/channels in"=w557, "error in"=w554) -> ("task out"=w549:refnum<k21>, "error out"=w544:errorcluster)  [unwired: 12 in]
          n153 = call <vilib>:"DAQmx Start Task.vi"("task/channels in"=w556, "error in"=w553) -> ("task out"=w548:refnum<k21>, "error out"=w543:errorcluster)  [unwired: 12 in]
          n154 = call <vilib>:"DAQmx Start Task.vi"("task/channels in"=w555, "error in"=w552) -> ("task out"=w547:refnum<k21>, "error out"=w542:errorcluster)  [unwired: 12 in]
        }
      }
      n155 = call <vilib>:"DAQmx Start Task.vi"("task/channels in"=w480, "error in"=w479) -> ("task out"=w459:refnum<k21>, "error out"=w338:errorcluster)  [unwired: 12 in]
      n156 = Build Array(w459, w366, w365) -> (w458:refnum<k21>[])
      n157 = Merge Errors(w338, w337, w336, w334, w333, w332, w329) -> (w335:errorcluster)
      n158 = Build Array(w364, w363, w362) -> (w361:refnum<k21>[])
    }
    frame 2 {
      w590 = tag "PXI_Clk10" ("RefClk.Src")
      w577 = 10123 items=["Finite Samples"=10178, "Continuous Samples"=10123] ("sample mode")
      # "master AI last"
      # "MASTER"
      n159 = Index Array(array=w654) -> (element #1=w679:T4, element #2=w641:T4)  [unwired: 2 in]
      n160 = Index Array(array=w629) -> (element #1=w628:T5, element #2=w607:T5)  [unwired: 2 in]
      n161 = Unbundle By Name(w679) -> ("AI.Min"=w652:dbl, "AI.Max"=w653:dbl, "Input physical channels"=w664:tag, "AI.Coupling"=w651:i32)
      n162 = Unbundle By Name(w641) -> ("AI.Min"=w648:dbl, "AI.Max"=w647:dbl, "Input physical channels"=w642:tag, "AI.Coupling"=w649:i32)
      n163 = Unbundle By Name(w628) -> ("AO.Min"=w625:dbl, "AO. Max"=w626:dbl, "Output physical channels"=w627:tag)
      n164 = Unbundle By Name(w607) -> ("AO.Min"=w610:dbl, "AO. Max"=w609:dbl, "Output physical channels"=w608:tag)
      n165 = call-poly <vilib>:"DAQmx Create Virtual Channel.vi"("maximum value"=w653, "minimum value"=w652, "input terminal configuration"=w564, "physical channels"=w664, "error in"=w569) -> ("task out"=w663:refnum<k21>, "error out"=w662:errorcluster)  [unwired: 9 in]
      n166 = call-poly <vilib>:"DAQmx Create Virtual Channel.vi"("maximum value"=w647, "minimum value"=w648, "input terminal configuration"=w564, "physical channels"=w642, "error in"=w569) -> ("task out"=w643:refnum<k21>, "error out"=w644:errorcluster)  [unwired: 9 in]
      n167 = call-poly <vilib>:"DAQmx Create Virtual Channel.vi"("maximum value"=w626, "minimum value"=w625, "output terminal configuration"=w565, "physical channels"=w627, "error in"=w569) -> ("task out"=w589:refnum<k21>, "error out"=w588:errorcluster)  [unwired: 9 in]
      n168 = call-poly <vilib>:"DAQmx Create Virtual Channel.vi"("maximum value"=w609, "minimum value"=w610, "output terminal configuration"=w565, "physical channels"=w608, "error in"=w569) -> ("task out"=w611:refnum<k21>, "error out"=w612:errorcluster)  [unwired: 9 in]
      n169 = Unbundle By Name(w579) -> ("#s"=w576:dbl, "Fs"=w578:dbl)
      n170 = property class="DAQmx Channel"(reference=w663, error in=w662, "AI.Coupling"=w651) -> (reference out=w661:refnum<k21>, error out=w660:errorcluster)
      n171 = property class="DAQmx Channel"(reference=w643, error in=w644, "AI.Coupling"=w649) -> (reference out=w645:refnum<k21>, error out=w646:errorcluster)
      n172 = Multiply(x=w657, y=w576) -> (x*y=w581:dbl)
      n173 = call <vilib>:"DAQmx Configure Input Buffer.vi"("task/channels in"=w661, "buffer size (in samples per channel)"=w581, "error in"=w660) -> ("task out"=w659:refnum<k21>, "error out"=w658:errorcluster)  [unwired: 11 in]
      n174 = call <vilib>:"DAQmx Configure Input Buffer.vi"("task/channels in"=w645, "buffer size (in samples per channel)"=w581, "error in"=w646) -> ("task out"=w640:refnum<k21>, "error out"=w639:errorcluster)  [unwired: 11 in]
      n175 = call-poly <vilib>:"DAQmx Timing.vi"("task/channels in"=w611, "sample mode"=w577, "samples per channel"=w576, "rate"=w578, "error in"=w612) -> ("task out"=w614:refnum<k21>, "error out"=w615:errorcluster)  [unwired: 9 in]
      n176 = call-poly <vilib>:"DAQmx Timing.vi"("task/channels in"=w659, "sample mode"=w577, "samples per channel"=w576, "rate"=w578, "error in"=w658) -> ("task out"=w678:refnum<k21>, "error out"=w650:errorcluster)  [unwired: 9 in]
      n177 = call-poly <vilib>:"DAQmx Timing.vi"("task/channels in"=w640, "sample mode"=w577, "samples per channel"=w576, "rate"=w578, "error in"=w639) -> ("task out"=w638:refnum<k21>, "error out"=w637:errorcluster)  [unwired: 9 in]
      n178 = call-poly <vilib>:"DAQmx Timing.vi"("task/channels in"=w589, "sample mode"=w577, "samples per channel"=w576, "rate"=w578, "error in"=w588) -> ("task out"=w623:refnum<k21>, "error out"=w622:errorcluster)  [unwired: 9 in]
      n179 = property class="DAQmx Timing" props=["More:Reference Clock:Source", "SampQuant.SampPerChan", "SampClk.Timebase.Rate", "SampClk.Timebase.Src"](reference=w678, error in=w650, "More:Reference Clock:Source"=w590) -> (reference out=w594:refnum<k21>, error out=w593:errorcluster, "SampQuant.SampPerChan"=w567:dbl, "SampClk.Timebase.Rate"=w566:dbl)  [unwired: 1 out]
      n180 = call "Get Terminal Name with Device Prefix.vi"("error in (no error)"=w593, "Local Terminal Name"="SyncPulse", "task/channels in"=w594) -> ("error out"=w673:errorcluster, "Terminal Name with Device Prefix"=w591:tag, "task out"=w674:refnum<k21>)  [unwired: 6 in]
      n181 = property class="DAQmx Timing"(reference=w638, error in=w637, "More:Reference Clock:Source"=w590, "More:Synchronization Pulse:Source"=w591) -> (reference out=w636:refnum<k21>, error out=w635:errorcluster)
      n182 = property class="DAQmx Timing"(reference=w623, error in=w622, "More:Reference Clock:Source"=w590, "More:Synchronization Pulse:Source"=w591) -> (reference out=w624:refnum<k21>, error out=w621:errorcluster)
      n183 = property class="DAQmx Timing"(reference=w614, error in=w615, "More:Reference Clock:Source"=w590, "More:Synchronization Pulse:Source"=w591) -> (reference out=w613:refnum<k21>, error out=w616:errorcluster)
      n184 = local write "SampQuant.SampPerChan"(w567) -> ()
      n185 = local write "SampClk.Timebase.Rate"(w566) -> ()
      n186 = call "Get Terminal Name with Device Prefix.vi"("error in (no error)"=w673, "Local Terminal Name"="ai/StartTrigger", "task/channels in"=w674) -> ("error out"=w671:errorcluster, "Terminal Name with Device Prefix"=w604:tag, "task out"=w672:refnum<k21>)  [unwired: 6 in]
      n187 = call-poly <vilib>:"DAQmx Trigger.vi"("task/channels in"=w636, "source"=w604, "error in"=w635) -> ("task out"=w634:refnum<k21>, "error out"=w633:errorcluster)  [unwired: 11 in]
      n188 = call-poly <vilib>:"DAQmx Trigger.vi"("task/channels in"=w624, "source"=w604, "error in"=w621) -> ("task out"=w620:refnum<k21>, "error out"=w619:errorcluster)  [unwired: 11 in]
      n189 = call-poly <vilib>:"DAQmx Trigger.vi"("task/channels in"=w613, "source"=w604, "error in"=w616) -> ("task out"=w617:refnum<k21>, "error out"=w618:errorcluster)  [unwired: 11 in]
      n190 = property class="DAQmx Timing"(reference=w672, error in=w671) -> (reference out=w668:refnum<k21>, error out=w669:errorcluster, "SyncPulse.SyncTime"=w670:dbl)
      n191 = property class="DAQmx Timing"(reference=w634, error in=w633) -> (reference out=w630:refnum<k21>, error out=w603:errorcluster, "SyncPulse.SyncTime"=w631:dbl)
      n192 = property class="DAQmx Timing"(reference=w620, error in=w619) -> (reference out=w602:refnum<k21>, error out=w600:errorcluster, "SyncPulse.SyncTime"=w606:dbl)
      n193 = property class="DAQmx Timing"(reference=w617, error in=w618) -> (reference out=w601:refnum<k21>, error out=w599:errorcluster, "SyncPulse.SyncTime"=w605:dbl)
      n194 = Build Array(w670, w631, w606, w605) -> (w667:dbl[])
      n195 = Array Max & Min(array=w667) -> (max value=w632:dbl)  [unwired: 3 out]
      n196 = property class="DAQmx Timing"(reference=w668, error in=w669, "SyncPulse.MinDelayToStart"=w632) -> (reference out=w665:refnum<k21>, error out=w666:errorcluster)
      n197 = call "4461 - Create AO waveforms.vi"("error in (no error)"=w569, "sampling info"=w579, "AO"=w580) -> ("error out"=w568:errorcluster, "AO Array"=w570:waveform(dbl)[])  [unwired: 5 in, 2 out]
      n198 = Index Array(array=w570) -> (element #1=w582:waveform(dbl), element #2=w587:waveform(dbl), element #3=w586:waveform(dbl), element #4=w585:waveform(dbl))  [unwired: 4 in]
      n199 = Build Array(w582, w587) -> (w584:waveform(dbl)[])
      n200 = Build Array(w586, w585) -> (w583:waveform(dbl)[])
      n201 = flat-sequence {
        tunnel: w666 -> [w707]
        tunnel: w665 -> [w708]
        tunnel: [w708] -> w696
        tunnel: [w707] -> w695
        tunnel: [w706] -> w694
        tunnel: w630 -> [w706]
        tunnel: [w705] -> w693
        tunnel: w603 -> [w705]
        tunnel: [w704] -> w692
        tunnel: w602 -> [w704]
        tunnel: [w700] -> w691
        tunnel: w601 -> [w701]
        tunnel: [w703] -> w690
        tunnel: w600 -> [w703]
        tunnel: w599 -> [w702]
        tunnel: [w699] -> w689
        tunnel: [w698] -> w688
        tunnel: w584 -> [w698]
        tunnel: w583 -> [w697]
        tunnel: [w719] -> w687
        tunnel: [w718] -> w686
        tunnel: w696 -> [w719]
        tunnel: w695 -> [w718]
        tunnel: [w717] -> w685
        tunnel: w694 -> [w717]
        tunnel: [w716] -> w684
        tunnel: w693 -> [w716]
        tunnel: [w712] -> w683
        tunnel: w692 -> [w713]
        tunnel: [w715] -> w682
        tunnel: w691 -> [w715]
        tunnel: [w711] -> w681
        tunnel: w690 -> [w710]
        tunnel: [w714] -> w680
        tunnel: w689 -> [w714]
        tunnel: w688 -> [w709]
        tunnel: [w733] -> w677
        tunnel: [w732] -> w676
        tunnel: w687 -> [w733]
        tunnel: w686 -> [w732]
        tunnel: w685 -> [w731]
        tunnel: w684 -> [w730]
        tunnel: w683 -> [w729]
        tunnel: w682 -> [w728]
        tunnel: w681 -> [w727]
        tunnel: w680 -> [w726]
        tunnel: [w725] -> w598
        tunnel: [w724] -> w597
        tunnel: [w723] -> w596
        tunnel: [w722] -> w574
        tunnel: [w721] -> w572
        tunnel: [w720] -> w571
        frame #0 {
          n202 = call-poly <vilib>:"DAQmx Write.vi"("task/channels in"=w701, "data"=w697, "error in"=w702) -> ("task out"=w700:refnum<k21>, "error out"=w699:errorcluster)  [unwired: 10 in, 1 out]
        }
        frame #1 {
          n203 = call-poly <vilib>:"DAQmx Write.vi"("task/channels in"=w713, "data"=w709, "error in"=w710) -> ("task out"=w712:refnum<k21>, "error out"=w711:errorcluster)  [unwired: 10 in, 1 out]
        }
        frame #2 {
          n204 = call <vilib>:"DAQmx Start Task.vi"("task/channels in"=w731, "error in"=w730) -> ("task out"=w725:refnum<k21>, "error out"=w722:errorcluster)  [unwired: 12 in]
          n205 = call <vilib>:"DAQmx Start Task.vi"("task/channels in"=w729, "error in"=w727) -> ("task out"=w724:refnum<k21>, "error out"=w721:errorcluster)  [unwired: 12 in]
          n206 = call <vilib>:"DAQmx Start Task.vi"("task/channels in"=w728, "error in"=w726) -> ("task out"=w723:refnum<k21>, "error out"=w720:errorcluster)  [unwired: 12 in]
        }
      }
      n207 = call <vilib>:"DAQmx Start Task.vi"("task/channels in"=w677, "error in"=w676) -> ("task out"=w656:refnum<k21>, "error out"=w575:errorcluster)  [unwired: 12 in]
      n208 = Build Array(w656, w598) -> (w655:refnum<k21>[])
      n209 = Merge Errors(w575, w574, w572, w571, w568) -> (w573:errorcluster)
      n210 = Build Array(w597, w596) -> (w595:refnum<k21>[])
    }
    frame 1 {
      w755 = tag "PXI_Clk10" ("RefClk.Src")
      w745 = 10123 items=["Finite Samples"=10178, "Continuous Samples"=10123] ("sample mode")
      # "master AI last"
      # "MASTER"
      n211 = Index Array(array=w782) -> (element=w807:T4)  [unwired: 1 in]
      n212 = Index Array(array=w776) -> (element=w775:T5)  [unwired: 1 in]
      n213 = Unbundle By Name(w807) -> ("AI.Min"=w780:dbl, "AI.Max"=w781:dbl, "Input physical channels"=w792:tag, "AI.Coupling"=w779:i32)
      n214 = Unbundle By Name(w775) -> ("AO.Min"=w772:dbl, "AO. Max"=w773:dbl, "Output physical channels"=w774:tag)
      n215 = call-poly <vilib>:"DAQmx Create Virtual Channel.vi"("maximum value"=w781, "minimum value"=w780, "input terminal configuration"=w735, "physical channels"=w792, "error in"=w739) -> ("task out"=w791:refnum<k21>, "error out"=w790:errorcluster)  [unwired: 9 in]
      n216 = call-poly <vilib>:"DAQmx Create Virtual Channel.vi"("maximum value"=w773, "minimum value"=w772, "output terminal configuration"=w734, "physical channels"=w774, "error in"=w739) -> ("task out"=w754:refnum<k21>, "error out"=w753:errorcluster)  [unwired: 9 in]
      n217 = Unbundle By Name(w747) -> ("#s"=w744:dbl, "Fs"=w746:dbl)
      n218 = property class="DAQmx Channel"(reference=w791, error in=w790, "AI.Coupling"=w779) -> (reference out=w789:refnum<k21>, error out=w788:errorcluster)
      n219 = Multiply(x=w785, y=w744) -> (x*y=w749:dbl)
      n220 = call <vilib>:"DAQmx Configure Input Buffer.vi"("task/channels in"=w789, "buffer size (in samples per channel)"=w749, "error in"=w788) -> ("task out"=w787:refnum<k21>, "error out"=w786:errorcluster)  [unwired: 11 in]
      n221 = call-poly <vilib>:"DAQmx Timing.vi"("task/channels in"=w787, "sample mode"=w745, "samples per channel"=w744, "rate"=w746, "error in"=w786) -> ("task out"=w806:refnum<k21>, "error out"=w778:errorcluster)  [unwired: 9 in]
      n222 = call-poly <vilib>:"DAQmx Timing.vi"("task/channels in"=w754, "sample mode"=w745, "samples per channel"=w744, "rate"=w746, "error in"=w753) -> ("task out"=w770:refnum<k21>, "error out"=w769:errorcluster)  [unwired: 9 in]
      n223 = property class="DAQmx Timing" props=["More:Reference Clock:Source", "SampQuant.SampPerChan", "SampClk.Timebase.Rate", "SampClk.Timebase.Src"](reference=w806, error in=w778, "More:Reference Clock:Source"=w755) -> (reference out=w759:refnum<k21>, error out=w758:errorcluster, "SampQuant.SampPerChan"=w737:dbl, "SampClk.Timebase.Rate"=w736:dbl)  [unwired: 1 out]
      n224 = call "Get Terminal Name with Device Prefix.vi"("error in (no error)"=w758, "Local Terminal Name"="SyncPulse", "task/channels in"=w759) -> ("error out"=w801:errorcluster, "Terminal Name with Device Prefix"=w756:tag, "task out"=w802:refnum<k21>)  [unwired: 6 in]
      n225 = property class="DAQmx Timing"(reference=w770, error in=w769, "More:Reference Clock:Source"=w755, "More:Synchronization Pulse:Source"=w756) -> (reference out=w771:refnum<k21>, error out=w768:errorcluster)
      n226 = local write "SampQuant.SampPerChan"(w737) -> ()
      n227 = local write "SampClk.Timebase.Rate"(w736) -> ()
      n228 = call "Get Terminal Name with Device Prefix.vi"("error in (no error)"=w801, "Local Terminal Name"="ai/StartTrigger", "task/channels in"=w802) -> ("error out"=w799:errorcluster, "Terminal Name with Device Prefix"=w764:tag, "task out"=w800:refnum<k21>)  [unwired: 6 in]
      n229 = call-poly <vilib>:"DAQmx Trigger.vi"("task/channels in"=w771, "source"=w764, "error in"=w768) -> ("task out"=w767:refnum<k21>, "error out"=w766:errorcluster)  [unwired: 11 in]
      n230 = property class="DAQmx Timing"(reference=w800, error in=w799) -> (reference out=w796:refnum<k21>, error out=w797:errorcluster, "SyncPulse.SyncTime"=w798:dbl)
      n231 = property class="DAQmx Timing"(reference=w767, error in=w766) -> (reference out=w763:refnum<k21>, error out=w762:errorcluster, "SyncPulse.SyncTime"=w765:dbl)
      n232 = Build Array(w798, w765) -> (w795:dbl[])
      n233 = Array Max & Min(array=w795) -> (max value=w777:dbl)  [unwired: 3 out]
      n234 = property class="DAQmx Timing"(reference=w796, error in=w797, "SyncPulse.MinDelayToStart"=w777) -> (reference out=w793:refnum<k21>, error out=w794:errorcluster)
      n235 = call "4461 - Create AO waveforms.vi"("error in (no error)"=w739, "sampling info"=w747, "AO"=w748) -> ("error out"=w738:errorcluster, "AO Array"=w740:waveform(dbl)[])  [unwired: 5 in, 2 out]
      n236 = Index Array(array=w740) -> (element #1=w750:waveform(dbl), element #2=w752:waveform(dbl))  [unwired: 2 in]
      n237 = Build Array(w750, w752) -> (w751:waveform(dbl)[])
      n238 = flat-sequence {
        tunnel: w794 -> [w820]
        tunnel: w793 -> [w821]
        tunnel: [w821] -> w816
        tunnel: [w820] -> w815
        tunnel: [w819] -> w814
        tunnel: w763 -> [w819]
        tunnel: [w818] -> w813
        tunnel: w762 -> [w818]
        tunnel: [w817] -> w812
        tunnel: w751 -> [w817]
        tunnel: [w828] -> w811
        tunnel: [w827] -> w810
        tunnel: w816 -> [w828]
        tunnel: w815 -> [w827]
        tunnel: [w825] -> w809
        tunnel: w814 -> [w826]
        tunnel: [w824] -> w808
        tunnel: w813 -> [w823]
        tunnel: w812 -> [w822]
        tunnel: [w834] -> w805
        tunnel: [w833] -> w804
        tunnel: w811 -> [w834]
        tunnel: w810 -> [w833]
        tunnel: w809 -> [w832]
        tunnel: w808 -> [w831]
        tunnel: [w830] -> w761
        tunnel: [w829] -> w741
        frame #0 {
        }
        frame #1 {
          n239 = call-poly <vilib>:"DAQmx Write.vi"("task/channels in"=w826, "data"=w822, "error in"=w823) -> ("task out"=w825:refnum<k21>, "error out"=w824:errorcluster)  [unwired: 10 in, 1 out]
        }
        frame #2 {
          n240 = call <vilib>:"DAQmx Start Task.vi"("task/channels in"=w832, "error in"=w831) -> ("task out"=w830:refnum<k21>, "error out"=w829:errorcluster)  [unwired: 12 in]
        }
      }
      n241 = call <vilib>:"DAQmx Start Task.vi"("task/channels in"=w805, "error in"=w804) -> ("task out"=w784:refnum<k21>, "error out"=w743:errorcluster)  [unwired: 12 in]
      n242 = Build Array(w784) -> (w783:refnum<k21>[])
      n243 = Merge Errors(w743, w741, w738) -> (w742:errorcluster)
      n244 = Build Array(w761) -> (w760:refnum<k21>[])
    }
  }
  "AI task" <- w14
  "AO Task" <- w12
  "error out" <- w6
  n245 = Initialize Array(0.0 ("element"), 8 ("dimension size")) -> (→"phase log":dbl[])
